vi "DPadMotorTest.vi"() -> ()   [LabVIEW 2024]
panel:
  in  "stop":bool
  in  "ddd":bool
  in  "dd":bool
  in  "d":bool
  in  "^\n^\n^":bool
  in  "^\n^":bool
  in  "^":bool
  in  "<<<":bool
  in  "<<":bool
  in  "<":bool
  in  ">>>":bool
  in  ">>":bool
  in  ">":bool
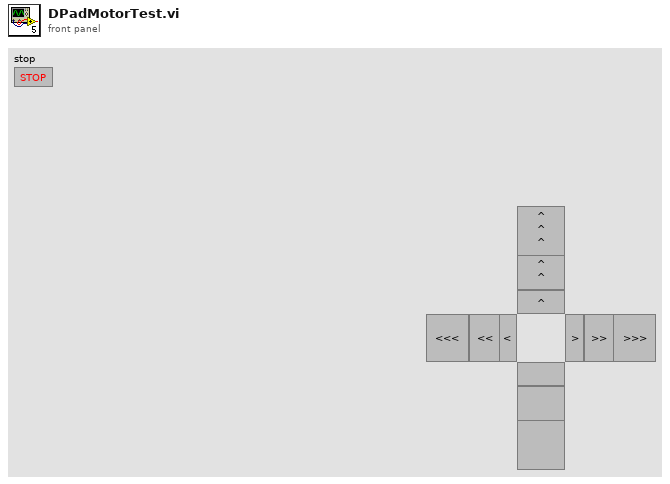
[diagram p1: front panel]
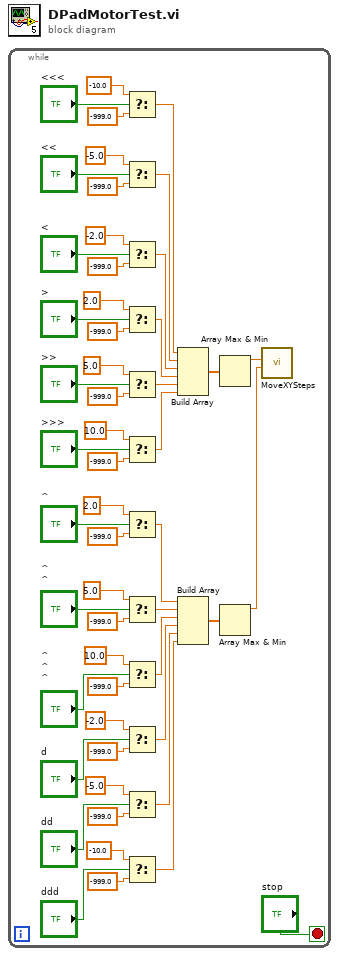
[diagram p0: block diagram]
diagram:
  n1 = while {
    stop <- "stop" stop-if-true
    n2 = Select(t=-10.0, s="<<<", f=-999.0) -> (s? t:f=w35:dbl)
    n3 = Select(t=-5.0, s="<<", f=-999.0) -> (s? t:f=w34:dbl)
    n4 = Select(t=-2.0, s="<", f=-999.0) -> (s? t:f=w33:dbl)
    n5 = Select(t=2.0, s=">", f=-999.0) -> (s? t:f=w32:dbl)
    n6 = Select(t=5.0, s=">>", f=-999.0) -> (s? t:f=w31:dbl)
    n7 = Select(t=10.0, s=">>>", f=-999.0) -> (s? t:f=w30:dbl)
    n8 = Select(t=2.0, s="^", f=-999.0) -> (s? t:f=w9:dbl)
    n9 = Select(t=5.0, s="^\n^", f=-999.0) -> (s? t:f=w8:dbl)
    n10 = Select(t=10.0, s="^\n^\n^", f=-999.0) -> (s? t:f=w7:dbl)
    n11 = Select(t=-2.0, s="d", f=-999.0) -> (s? t:f=w4:dbl)
    n12 = Select(t=-5.0, s="dd", f=-999.0) -> (s? t:f=w5:dbl)
    n13 = Select(t=-10.0, s="ddd", f=-999.0) -> (s? t:f=w6:dbl)
    n14 = Build Array(w35, w34, w33, w32, w31, w30) -> (w29:dbl[])
    n15 = Build Array(w9, w8, w7, w4, w5, w6) -> (w3:dbl[])
    n16 = Array Max & Min(array=w29) -> (max value=w28:dbl)  [unwired: 3 out]
    n17 = Array Max & Min(array=w3) -> (max value=w2:dbl)  [unwired: 3 out]
    n18 = call "MoveXYSteps.vi"("Y Steps"=w2, "X Steps"=w28) -> ()  [unwired: 9 in, 1 out]
  }
